vi "ChannelList_GetNames.vi"(8 "error in (no error)":errorcluster, 11 "OXY_SCPI Reseource In":refnum<visa-resource-name>) -> (0 "error out":errorcluster, 1 "communication_data":T1, 2 "Channel List":T2[](array[typedef]), 3 "OXY_SCPI Reseource Out":refnum<visa-resource-name>)   [LabVIEW 2018, in "OXYGEN.lvlib"]
doc: "Queries the name and ids of all channels."
uses:
  OXYGEN.lvlib
  TypeDefs/Cluster_ChannelList_Names.ctl
  TypeDefs/Cluster_RawCommData.ctl
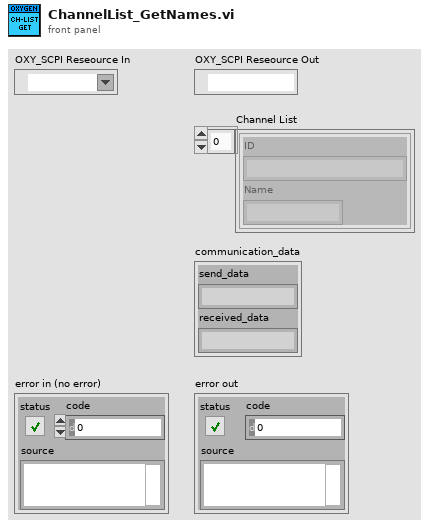
[diagram p1: front panel]
types:
  T1 = typedef "OXYGEN.lvlib/Cluster_RawCommData.ctl" = cluster{"send_data":string, "received_data":string}
  T2 = typedef "OXYGEN.lvlib/Cluster_ChannelList_Names.ctl" = cluster{"ID":string, "Name":string}
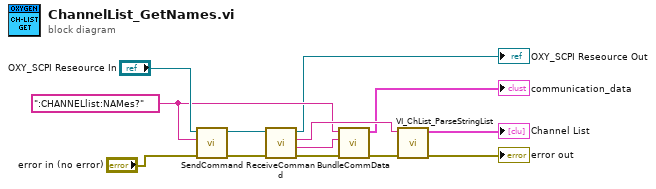
[diagram p0: block diagram]
diagram:
  w4 = ":CHANNELlist:NAMes?"
  n1 = call "SendCommand.vi"("error in (no error)"="error in (no error)", "String to Send"=w4, "OXY_SCPI Reseource In"="OXY_SCPI Reseource In") -> ("error out"=w13:errorcluster, "OXY_SCPI Reseource Out"=w12:refnum<visa-resource-name>)  [unwired: 7 in]
  n2 = call "ReceiveCommand.vi"("error in (no error)"=w13, "OXY_SCPI Reseource In"=w12) -> ("error out"=w10:errorcluster, "received Data with Header"=w6:string, "received Data"=w5:string, "OXY_SCPI Reseource Out"=→"OXY_SCPI Reseource Out":refnum<visa-resource-name>)  [unwired: 6 in]
  n3 = call "BundleCommData.vi"("error in (no error)"=w10, "received_data"=w6, "send_data"=w4) -> ("error out"=w9:errorcluster, "communication_data"=→"communication_data":T1)  [unwired: 7 in]
  n4 = call "VI_ChList_ParseStringList.vi"("error in (no error)"=w9, "ChList_RawString"=w5) -> ("error out"=→"error out":errorcluster, "Channel List"=→"Channel List":cluster{"ID":string, "Name":string}[])  [unwired: 8 in]
